vi "mxwScript_API_SetVal_GenerateSubVI.vi"(8 "error in (no error)":errorcluster, 11 "CodeGenRecipe":T2) -> (0 "error out":errorcluster, 3 "parameter":T1)   [LabVIEW 2017]
uses:
  codeGenAPISupport.llb/cgAPI_mxwCodeGenCompleteRecipe.ctl
  codeGenAPISupport.llb/cgAPI_mxwScript_TemplateInfo.ctl
  codeGenAPISupport.llb/cgAPI_mxwScript_Wire_InputWireConnection.ctl
  codeGenAPISupport.llb/cgAPI_mxwScript_Parameter.ctl
  codeGenAPISupport.llb/cgAPI_mxwScript_ConnPaneConnectionSpec.ctl
  codeGenAPISupport.llb/cgAPI_mxwScript_OptionData.ctl
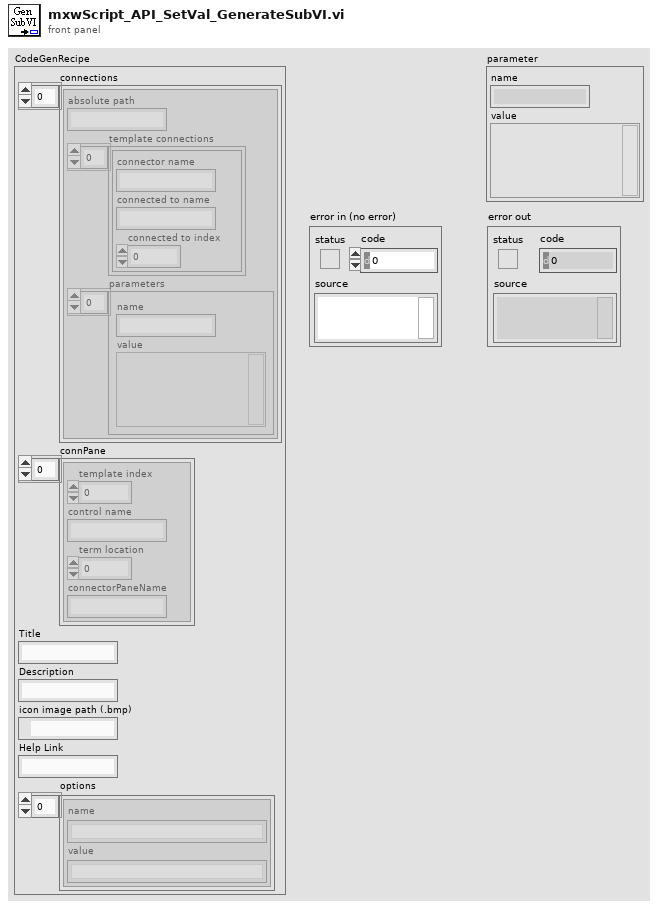
[diagram p1: front panel]
types:
  T1 = typedef "cgAPI_mxwScript_Parameter.ctl" = cluster{"name":string, "value":variant}
  T2 = typedef "cgAPI_mxwCodeGenCompleteRecipe.ctl" = cluster{"connections":T3[], "connPane":T5[], "Title":string, "Description":string, "icon image path (.bmp)":path, "Help Link":string, "options":T6[]}
  T3 = typedef "cgAPI_mxwScript_TemplateInfo.ctl" = cluster{"absolute path":string, "template connections":T4[], "parameters":T1[]}
  T4 = typedef "cgAPI_mxwScript_Wire_InputWireConnection.ctl" = cluster{"connector name":string, "connected to name":string, "connected to index":i32}
  T5 = typedef "cgAPI_mxwScript_ConnPaneConnectionSpec.ctl" = cluster{"template index":u32, "control name":string, "term location":i32, "connectorPaneName":string}
  T6 = typedef "cgAPI_mxwScript_OptionData.ctl" = cluster{"name":string, "value":string}
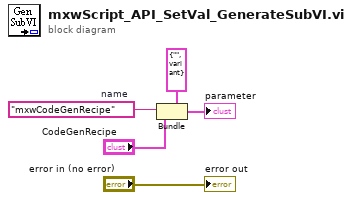
[diagram p0: block diagram]
diagram:
  w1 = "mxwCodeGenRecipe"  # name
  n1 = Bundle(cluster=T1 {"name"="", "value"=variant} ("parameter"), "name"=w1, "value"="CodeGenRecipe") -> (→"parameter":T1)
  "error out" <- "error in (no error)"
